vi "Stop Core.vi"(10 "final error code":i32, 11 "TCP_Server_Connection_Handler in":refnum<class "TCP_Server_Connection_Handler.lvclass">) -> (3 "TCP_Server_Connection_Handler out":refnum<class "TCP_Server_Connection_Handler.lvclass">)   [LabVIEW 2023, in "TCP_Server_Connection_Handler.lvlib" / "TCP_Server_Connection_Handler.lvclass"]
doc: "(<B>Filename</B>: Actor Framework.lvlib:Actor.lvclass:Stop Core.vi)\n\nDefines what the actor does before it stops. Use the <B>final error code</B> input to determine whether the actor shut down in response to an error.\n\nBy default, this method passes the Stop message along to all auto-stop nested actors. A descendant class may override this method to define additional behavior, such as shutting down any processes the actor initiated in its override of the Actor Core method."
uses:
  TCP_Server_Connection_Handler.lvclass
  TCP_Server_Connection_Handler.lvclass/TCP_Server_Connection_Handler.ctl
  <vilib>/ActorFramework/Actor/Actor.lvclass/Actor.ctl
  TCP_Connections_Controller Messages/ConnectionClosed Msg/ConnectionClosed Msg.lvclass/ConnectionClosed Msg.ctl
  <vilib>/ActorFramework/Message Enqueuer/Message Enqueuer.lvclass/Message Enqueuer.ctl
  d81dd845-ac8b-4d1a-8674-86199b1a0b2c.vi
  <vilib>/ActorFramework/Message Enqueuer/Enqueue.vi
  TCP_Connections_Controller Messages/ConnectionClosed Msg/ConnectionClosed Msg.lvclass
  <vilib>/ActorFramework/Message Priority Queue/Priority Enqueue.vi
  <vilib>/ActorFramework/Actor/Actor.lvclass
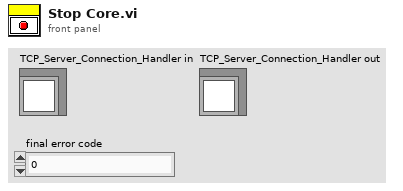
[diagram p1: front panel]
types:
  T1 = typedef "TCP_Listener.lvlib/ConnectionInformation.ctl" = cluster{"Connection number":i32, "Remote Address":string, "Remote Port":u16, "Connection ID":refnum<k5>}
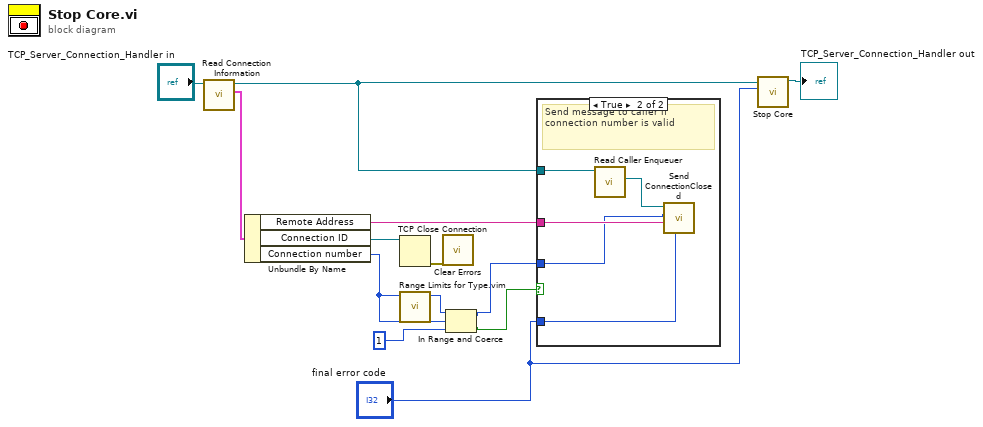
[diagram p0: block diagram]
diagram:
  n1 = call "Read Connection Information.vi"("TCP_Server_Connection_Handler in"="TCP_Server_Connection_Handler in") -> ("Connection Information"=w11:T1, "TCP_Server_Connection_Handler out"=w8:refnum<class "TCP_Server_Connection_Handler.lvclass">)  [unwired: 8 in, 1 out]
  n2 = Unbundle By Name(w11) -> ("Remote Address"=w10:string, "Connection ID"=w9:refnum<k5>, "Connection number"=w2:i32)
  n3 = TCP Close Connection(connection ID=w9) -> (error out=w1:errorcluster)  [unwired: 2 in, 1 out]
  n4 = call "Range Limits for Type.vim"("type"=w2) -> ("maximum value for type"=w6:i32)  [unwired: 9 in, 1 out]
  n5 = call <vilib>:"Clear Errors.vi"("error in (no error)"=w1) -> ()  [unwired: 5 in, 2 out]
  n6 = In Range and Coerce(upper limit=w6, x=w2, lower limit=1) -> (coerced(x)=w4:i32, In Range?=w5:bool)
  n7 = case shown="True" w5 {
    tunnel: w8 -> [_ w17]
    tunnel: w10 -> [_ w16]
    tunnel: "final error code" -> [_ w15]
    tunnel: w4 -> [_ w14]
    frame False {
    }
    frame True {
      # "Send message to caller if connection number is valid"
      n8 = call <vilib>:"Read Caller Enqueuer.vi"("Actor"=w17) -> ("Caller Enqueuer"=w18:refnum<class "Message Enqueuer.lvclass">)  [unwired: 10 in]
      n9 = call "Send ConnectionClosed.vi"("FinaErrorCode"=w15, "ClientIP"=w16, "ConnectionNumber"=w14, "Message Enqueuer"=w18) -> ()  [unwired: 6 in, 2 out]
    }
  }
  n10 = call-parent "Stop Core.vi"("final error code"="final error code", "Actor in"=w8) -> ("Actor out"=→"TCP_Server_Connection_Handler out":refnum<class "TCP_Server_Connection_Handler.lvclass">)  [unwired: 9 in]
